vi "Left To Cargo From Hab 1.vi"   [LabVIEW 2018]
uses:
  Support Code/Path Data.ctl
  Framework/Robot Global Data.vi
types:
  T1 = typedef "Path Data.ctl" = cluster{"Maneuver":enum16{"MAX 90", "MAX 180", "Turn to Home", "Turn to Rocket", "Auto-Align", "Turn to ..."}, "Rotation Direction":enum16{"N/A", "Right", "Left"}}[]
  T2 = typedef "Command Status Info.ctl" = cluster{"Name":string, "Status":T3, "notifier out":T4}
  T3 = typedef "Completion Status.ctl" = enum16{"Successful", "Aborted", "Incomplete"}
  T4 = typedef "Completion Notifier.ctl" = refnum<notifier>
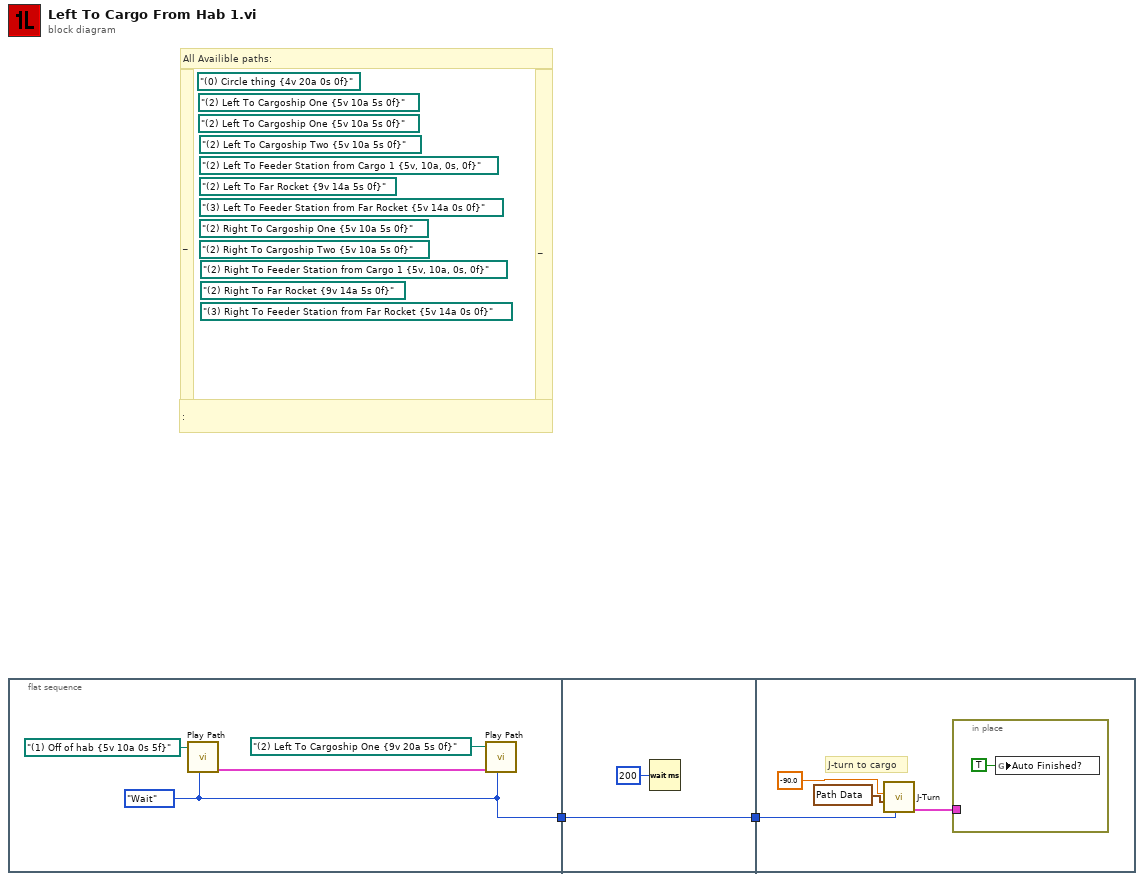
[diagram p0: block diagram]
diagram:
  (unwired) path "(3) Right To Feeder Station from Far Rocket {5v 14a 0s 0f}"
  (unwired) path "(2) Right To Far Rocket {9v 14a 5s 0f}"
  (unwired) path "(2) Right To Feeder Station from Cargo 1 {5v, 10a, 0s, 0f}"
  (unwired) path "(2) Right To Cargoship Two {5v 10a 5s 0f}"
  (unwired) path "(2) Right To Cargoship One {5v 10a 5s 0f}"
  (unwired) path "(3) Left To Feeder Station from Far Rocket {5v 14a 0s 0f}"
  (unwired) path "(2) Left To Far Rocket {9v 14a 5s 0f}"
  (unwired) path "(2) Left To Feeder Station from Cargo 1 {5v, 10a, 0s, 0f}"
  (unwired) path "(2) Left To Cargoship Two {5v 10a 5s 0f}"
  (unwired) path "(2) Left To Cargoship One {5v 10a 5s 0f}"
  (unwired) path "(2) Left To Cargoship One {5v 10a 5s 0f}"
  (unwired) path "(0) Circle thing {4v 20a 0s 0f}"
  # ":"
  # "_"
  # "_"
  # "All Availible paths:"
  n1 = flat-sequence {
    tunnel: [w3] -> w1
    tunnel: [w7] -> w2
    tunnel: w1 -> [w7]
    tunnel: w2 -> [w9]
    frame #0 {
      w3 = enum16{"Start", "Wait"}."Wait" ("Synchronication")
      n2 = call "Play Path.vi"("Synchronication"=w3, "Path"=path "(1) Off of hab {5v 10a 0s 5f}") -> ("Command Info Out"=w6:T2)  [unwired: 9 in]
      n3 = call "Play Path.vi"("Synchronication"=w3, "Command Info In"=w6, "Path"=path "(2) Left To Cargoship One {9v 20a 5s 0f}") -> ()  [unwired: 8 in, 1 out]
    }
    frame #1 {
      n4 = Wait (ms)(milliseconds to wait=u32 200) -> ()  [unwired: 1 out]
    }
    frame #2 {
      # "J-turn to cargo"
      n5 = call "J-Turn.vi"("Synchronication"=w9, "Path Data"=T1 [{"Maneuver"=enum."Turn to ...", "Rotation Direction"=enum."N/A"}, {"Maneuver"=enum."MAX 90", "Rotation Direction"=enum."N/A"}, {"Maneuver"=enum."MAX 90", "Rotation Direction"=enum."N/A"}], "Angle boi"=-90.0) -> ("Command Info Out"=w12:T2)  [unwired: 8 in]
      n6 = in-place {
        in-place-border: w12 -> [_]
        n7 = global write "Robot Global Data.vi" "Auto Finished?"(TRUE ("Auto Finished?")) -> ()
      }
    }
  }
